vi "runtest Pre-Process Test.vi"(6 "Username (\"\")":string, 7 "Fields In":T1[](array[typedef]), 8 "error in (no error)":errorcluster, 10 "Test Configuration (\"\")":string, 11 "Test_ID (\"\")":string) -> (0 "error out":errorcluster, 1 "Files Found?":bool, 2 "New Test Configuration":string, 3 "Test_ID Out":string, 5 "Fields Out":T1[](array[typedef]))   [LabVIEW 2011]
uses:
  server/database/Fields/Field Record.ctl
  server/database/Fields/Field DataTypes.ctl
  server/database/Fields/Field NextItem.ctl
  tests/Test Function.ctl
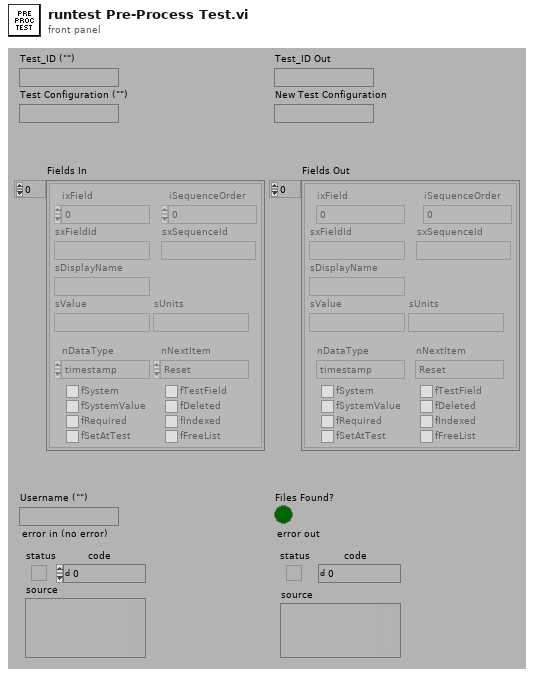
[diagram p1: front panel]
types:
  T1 = typedef "Field Record.ctl" = cluster{"ixField":i32, "iSequenceOrder":i32, "sxFieldId":string, "sxSequenceId":string, "sDisplayName":string, "sValue":string, "sUnits":string, "nDataType":T2, "nNextItem":T3, "fSystem":bool, "fSystemValue":bool, "fRequired":bool, "fSetAtTest":bool, "fTestField":bool, "fDeleted":bool, "fIndexed":bool, "fFreeList":bool}
  T2 = typedef "Field DataTypes.ctl" = enum32{"text", "numeric", "list", "timestamp", "boolean"}
  T3 = typedef "Field NextItem.ctl" = enum32{"Reset", "Retain", "Auto-Increment"}
  T4 = typedef "Test Function.ctl" = enum16{"Test Config", "Test Storage", "Test Pre-Process", "Unflatten Test Parameters", "Flatten Test Parameters"}
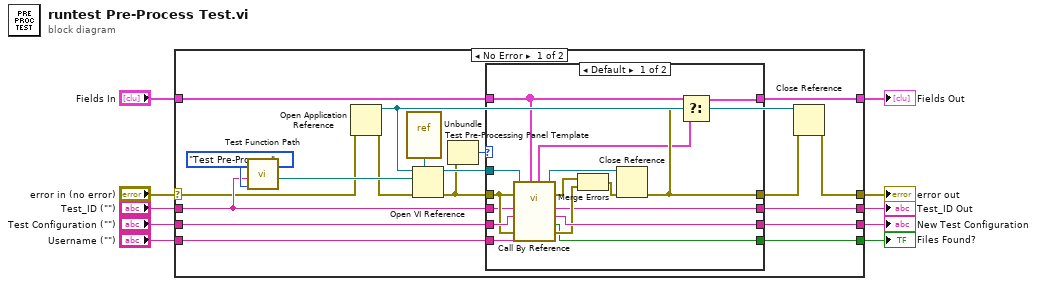
[diagram p0: block diagram]
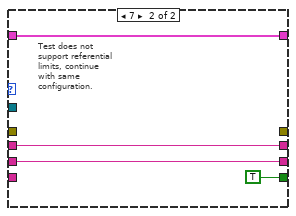
[diagram p2: hidden frame]
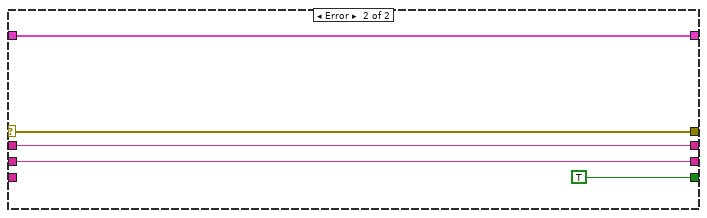
[diagram p3: hidden frame]
diagram:
  n1 = case shown="No Error" "error in (no error)" {
    selector: "error in (no error)" -> [w13 w52]
    tunnel: "Test Configuration (\"\")" -> [w25 w50]
    tunnel: [w24 w50] -> w9
    tunnel: "Fields In" -> [w23 w53]
    tunnel: [w22 w53] -> w7
    tunnel: "Username (\"\")" -> [w21 _]
    tunnel: [w15 w52] -> w5
    tunnel: "Test_ID (\"\")" -> [w18 w51]
    tunnel: [w17 w51] -> w3
    tunnel: [w16 TRUE ("Files Found?")] -> w1
    frame No Error {
      n2 = call "Test Function Path.vi"("Object Type (Test Config)"=Test_Function."Test Pre-Process", "Object Name (\"\")"=w18) -> ("Object Path"=w27:path)  [unwired: 1 in, 8 out]
      n3 = Open Application Reference(8:w13) -> (0:w12:errorcluster, 3:w11:refnum<vi>)  [unwired: 3 in]
      n4 = vi-ref "Test Pre-Processing Panel Template.vi"() -> ("vi reference"=w28:refnum<vi>)
      n5 = Open VI Reference(type specifier VI Refnum (for type only)=w28, application reference (local)=w11, vi path=w27, error in (no error)=w12) -> (vi reference=w26:refnum<vi>, error out=w19:errorcluster)  [unwired: 1 in, 1 out]
      n6 = Unbundle(w19) -> ("code"=w20:i32)  [unwired: 2 out]
      n7 = case shown="Default" w20 {
        tunnel: w26 -> [w44 _]
        tunnel: w25 -> [w43 w48]
        tunnel: [w42 w48] -> w24
        tunnel: w18 -> [w31 w46]
        tunnel: w23 -> [w34 w47]
        tunnel: [w32 w47] -> w22
        tunnel: w21 -> [w39 _]
        tunnel: [w35 _] -> w14
        tunnel: w19 -> [w36 _]
        tunnel: [w31 w46] -> w17
        tunnel: [w30 TRUE ("Files Found?")] -> w16
        frame Default {
          n8 = call-by-ref "?"(reference=w44, error in=w36, "Username (\"\")"=w39, "Fields In"=w34, "error in (no error)"=w36, "Test Configuration (\"\")"=w43, "Test_ID (\"\")"=w31) -> (reference out=w38:refnum<vi>, error out=w41:errorcluster, 0:"error out"=w40:errorcluster, "Files Found?"=w30:bool, "New Test Configuration"=w42:string, "Fields Out"=w33:T1[])  [unwired: 2 in, 1 out]
          n9 = Merge Errors(w41, w40) -> (w37:errorcluster)
          n10 = Close Reference(reference=w38, error in (no error)=w37) -> (error out=w35:errorcluster)
          n11 = Select(t=w34, s=w35, f=w33) -> (s? t:f=w32:T1[])
        }
        frame 7 {
          # "Test does not\nsupport referential\nlimits, continue\nwith same\nconfiguration."
        }
      }
      n12 = Close Reference(reference=w11, error in (no error)=w14) -> (error out=w15:errorcluster)
    }
    frame Error {
    }
  }
  "error out" <- w5
  "New Test Configuration" <- w9
  "Test_ID Out" <- w3
  "Fields Out" <- w7
  "Files Found?" <- w1
